vi "LuaVIEW Get Task State Reference.vi"(5 "LuaVIEW reference in":T2, 11 "error in (no error)":errorcluster) -> (4 "task state reference":T1, 6 "LuaVIEW reference out":T2, 15 "error out":errorcluster)   [LabVIEW 2012]
doc: "Returns a reference to the task state object when the LuaVIEW state is part of a task context. Otherwise an error is returned. This VI is used by LuaVIEW functions that operate on the task state of the calling context."
uses:
  typedefs/t_LuaVIEW Task State Pane.ctl
  typedefs/t_LuaVIEW Reference.ctl
  typedefs/et_LuaVIEW CIN Actions.ctl
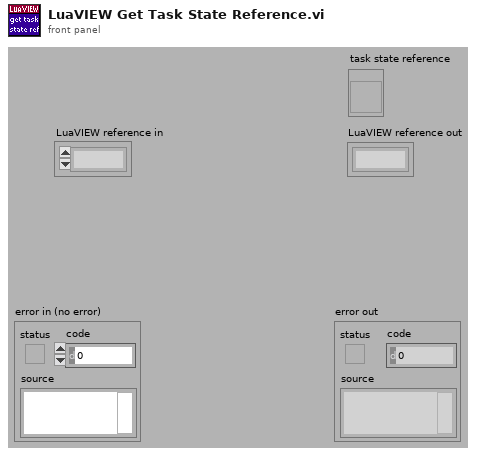
[diagram p1: front panel]
types:
  T1 = typedef "t_LuaVIEW Task State Pane.ctl" = refnum<vi>
  T2 = typedef "t_LuaVIEW Reference.ctl" = refnum<k1>
  T3 = typedef "et_LuaVIEW CIN Actions.ctl" = enum16{"checksynopsis", "_open", "_registerpublic", "_registerexport", "__never_an_error_result_ns", "luaversion", "cinversion", "_totals", "_taskcount", "pathological", "_unregnextpublic", "registryusecount", "__per_state_actions", "regsetprivate", "regsetindex", "regsetmodule", "_revokeexports", "_usepublic", "prepare", "compile", "execute", "call", "unregstaterefs", "_close", "pullboolean", "pullnumber", "pullI8", "pullU8", "pullI16", "pullU16", "pullI32", "pullU32", "pullobject", "pullrefnum", "pullstring", "pullflat", "pushflat", "pushobject", "getattribute", "setattribute", "stacktostring", "_startyieldtest", "_endyieldtest", "_pollprintbuffer", "__never_an_error_result_ps", "_pollexport", "setclone", "forcecleanup", "gettop", "clearstack", "insert", "pushboolean", "pushnumber", "pushrefnum", "pushstring", "pushnil", "pushvalue", "gettaskref", "settaskref"}
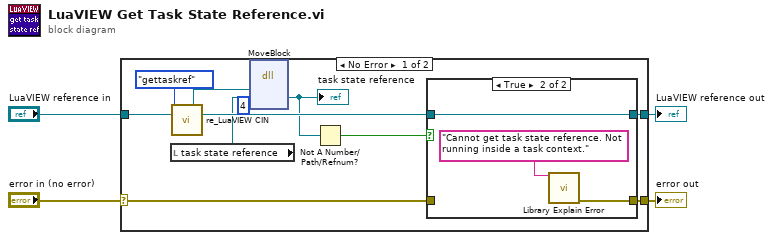
[diagram p0: block diagram]
diagram:
  n1 = case shown="No Error" "error in (no error)" {
    selector: "error in (no error)" -> [w11 w22]
    tunnel: [w12 w21] -> w4
    tunnel: [w10 w22] -> w3
    tunnel: "LuaVIEW reference in" -> [w14 w21]
    frame No Error {
      n2 = local read "task state reference"() -> (w7:T1)
      n3 = call "re_LuaVIEW CIN.vi"("action"=et_LuaVIEW_CIN_Actions."gettaskref", "LuaVIEW reference in"=w14) -> ("refnum out"=w8:refnum<vi>, "LuaVIEW reference out"=w13:T2)  [unwired: 7 in, 5 out]
      n4 = dll-call lib="LabVIEW" fn="MoveBlock"("refnum out"=w8, "task state reference"=w7, "len"=4) -> ("task state reference"=w6:T1)  [unwired: 6 in, 2 out]
      "task state reference" <- w6
      n5 = Not A Number/Path/Refnum?(number/path/refnum=w6) -> (NaN/Path/Refnum?=w9:bool)
      n6 = case shown="True" w9 {
        tunnel: w13 -> [w17 w20]
        tunnel: [w17 w20] -> w12
        tunnel: [w16 w19] -> w10
        tunnel: w11 -> [w16 _]
        frame False {
        }
        frame True {
          n7 = call "Library Explain Error.vi"("explanation prefix (none)"="Cannot get task state reference. Not running inside a task context." ("string out")) -> ("explained error"=w19:errorcluster)  [unwired: 14 in]
        }
      }
    }
    frame Error {
    }
  }
  "LuaVIEW reference out" <- w4
  "error out" <- w3
